vi "loadMSTReleaseFormNew.vi"() -> ()   [LabVIEW 2012]
uses:
  <vilib>/Utility/NIReport.llb/NI_report.lvclass
  <vilib>/addons/database/Connection.llb/DB Tools Open Connec (Path).vi
  <vilib>/addons/_office/excel.llb/Excel Get Data (str).vi
  <vilib>/addons/database/Connection.llb/Conn Execute.vi
  <vilib>/addons/database/Recordset.llb/Rec Fetch Integer Data (R).vi
  <vilib>/addons/database/Recordset.llb/Rec Destroy - Connection.vi
  <vilib>/Utility/NIReport.llb/Excel/NI_Excel.lvclass
  <vilib>/addons/_office/NI_ReportGenerationToolkit.lvlib
  <vilib>/addons/database/NI_Database_API.lvlib
panel:
  out "data 2":i32
  out "appended path 4":path
  out "appended path 3":path
  out "concatenated string 3":string
  out "error out 3":errorcluster
  out "row":i32
  out "concatenated string 2":string
  out "appended path 2":path
  out "data":string
  in  "start (0, 0)":cluster{"start row":i32, "start column":i32}
  out "PCB":string
  out "TestProgram":string
  out "Temp":string
  out "Product":string
  out "x+y":dbl
  out "String":string
  out "error out":errorcluster
  out "concatenated string":string
  out "error out 4":errorcluster
  out "appended path":path
  out "error out 2":errorcluster
  in  "path":path=path "O:/Monitor/Recipe/MST"
  out "filenames":string[](array[string])
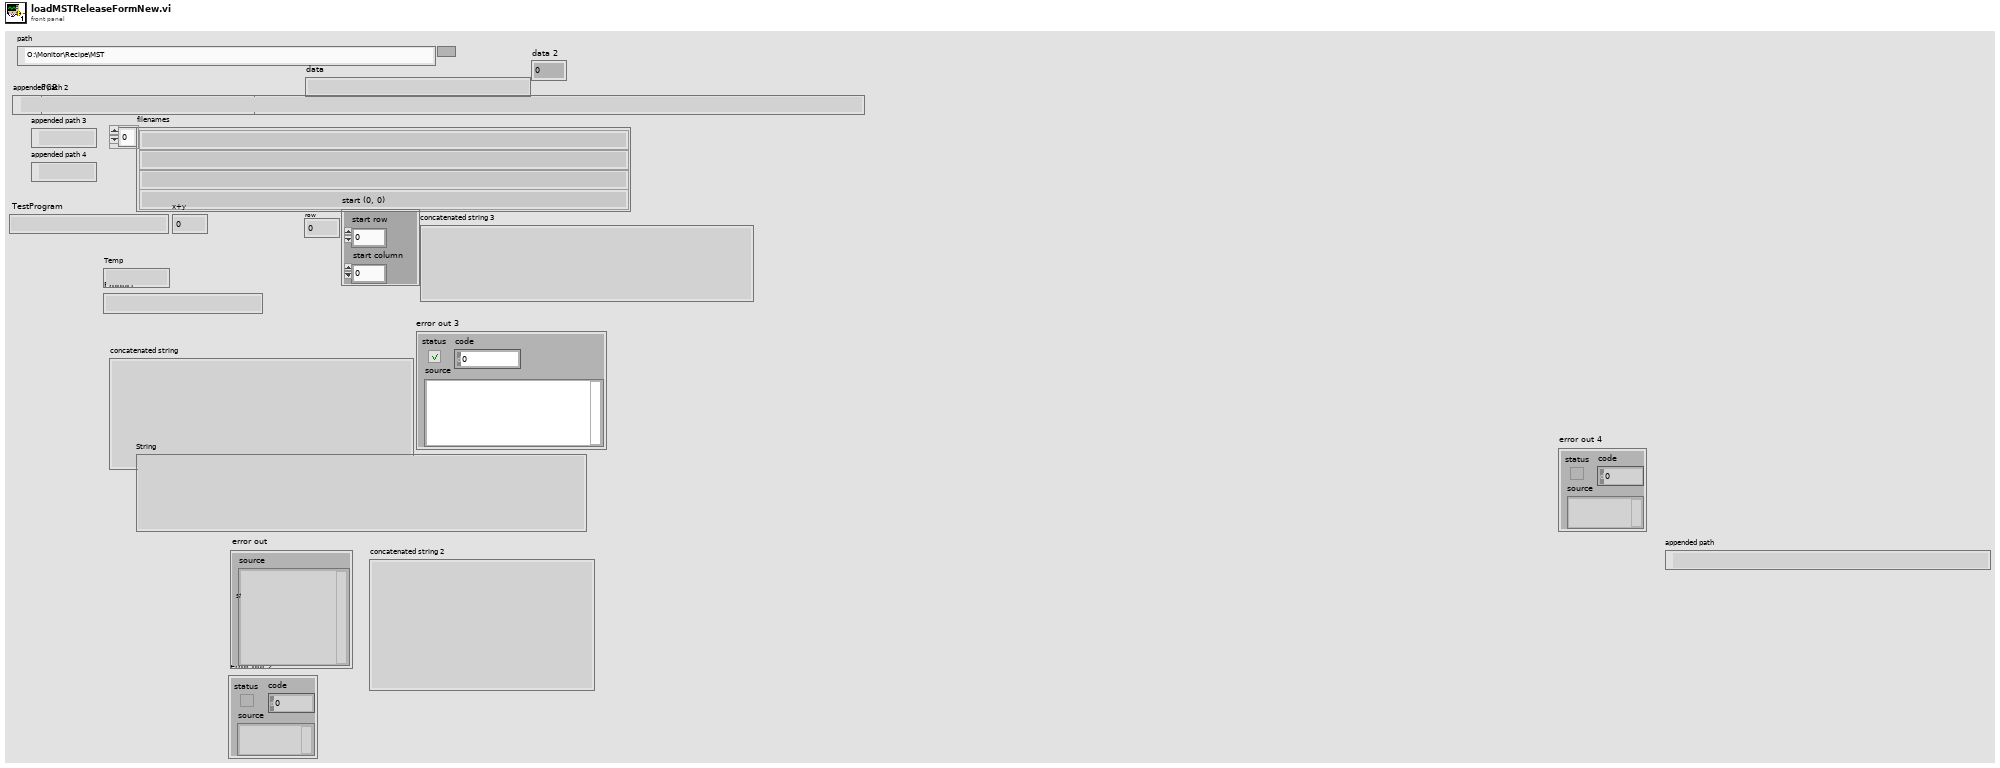
[diagram p1: front panel]
types:
  T1 = enum16{"Standard Report", "HTML", "Word", "Excel"}
  T2 = typedef "NI_Database_API.lvlib/Conn ObjectReference.ctl" = refnum<k1>
  T3 = typedef "NI_Database_API.lvlib/Rec ObjectReference.ctl" = refnum<k1>
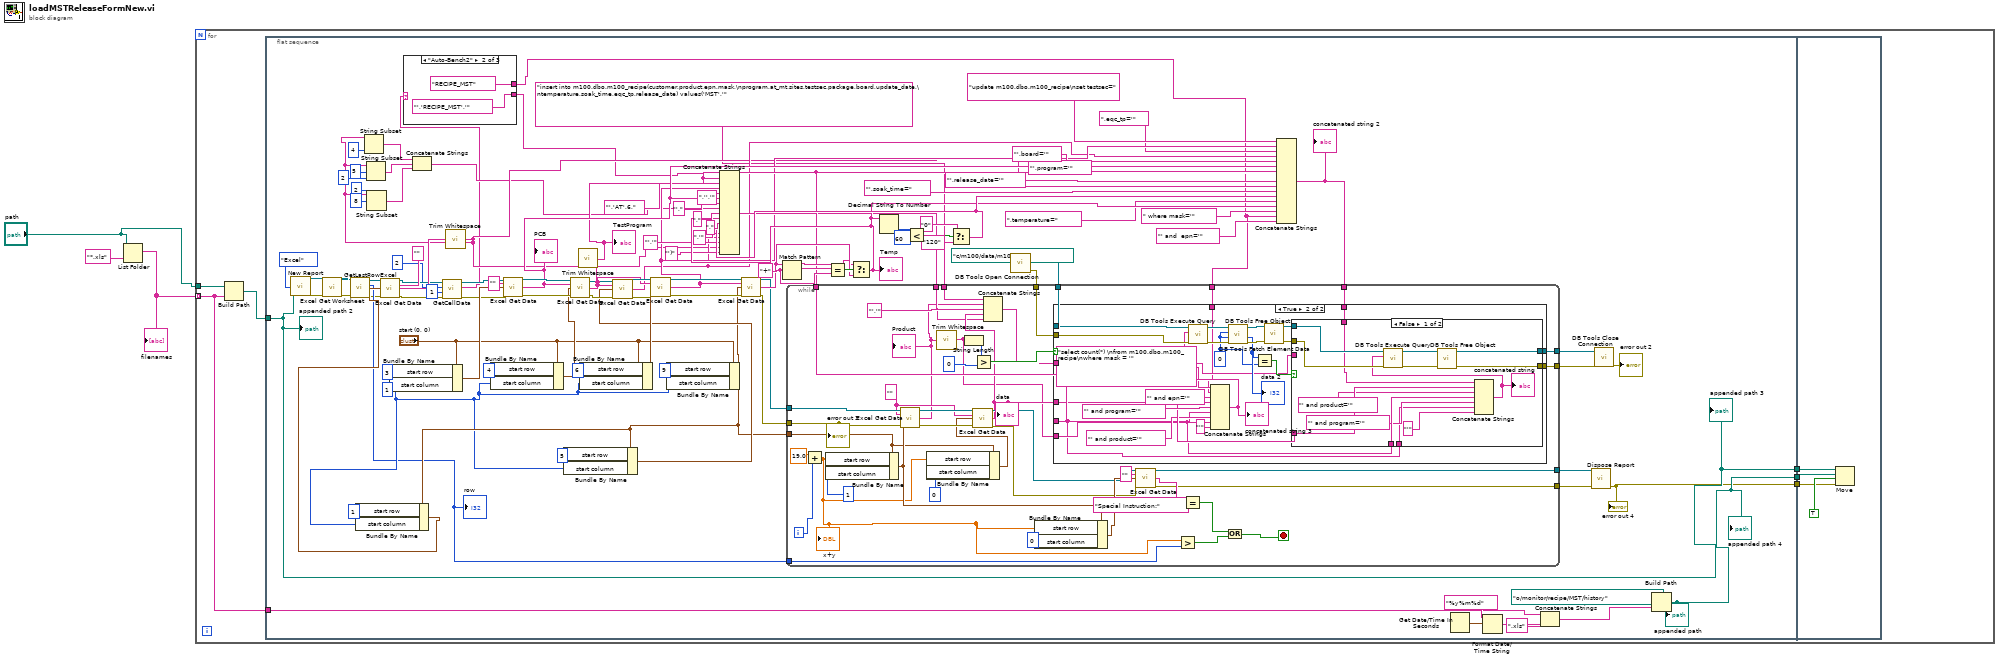
[diagram p0: block diagram]
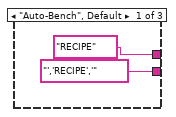
[diagram p2: hidden frame]
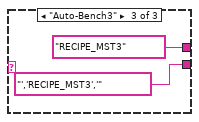
[diagram p3: hidden frame]
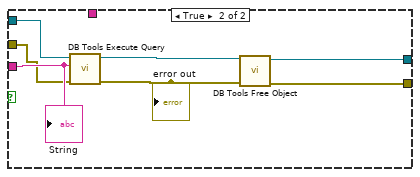
[diagram p5: hidden frame]
diagram:
  n1 = List Folder(path="path", pattern="*.xls") -> (filenames=w1:string[])  [unwired: 2 in, 3 out]
  "filenames" <- w1
  n2 = for {
    tunnel: "path" -> [w9]
    tunnel: w1 -> [w8] mode=indexing
    n3 = Build Path(base path=w9, name or relative path=w8) -> (appended path=w5:path)
    n4 = flat-sequence {
      tunnel: w8 -> [w74]
      tunnel: [w35] -> w7
      tunnel: [w34] -> w6
      tunnel: w5 -> [w34]
      tunnel: [w23] -> w4
      tunnel: w7 -> [w218]
      tunnel: w6 -> [w219]
      tunnel: w4 -> [w216]
      frame #0 {
        w101 = "+" ("regular expression")
        w48 = 1 ("start column")
        n5 = call <vilib>:"New Report.vi"("report type"=T1."Excel" ("Report Type"), "template (empty)"=w34) -> ("report out"=w117:refnum<class "NI_report.lvclass">, "error out"=w116:errorcluster)  [unwired: 12 in]
        n6 = call <vilib>:"Excel Get Worksheet.vi"("report in"=w117, "error in (no error)"=w116) -> ("report out"=w42:refnum<class "NI_report.lvclass">, "error out"=w43:errorcluster)  [unwired: 12 in]
        n7 = call "GetLastRowExcel.vi"("error in (no error)"=w43, "report in"=w42) -> ("error out"=w21:errorcluster, "row"=w40:i32, "report out"=w41:refnum<class "NI_report.lvclass">)  [unwired: 7 in]
        "row" <- w40
        n8 = Bundle By Name(cluster="start (0, 0)", "start row"=3, "start column"=w48) -> (w115:cluster{"start row":i32, "start column":i32})
        n9 = Bundle By Name(cluster="start (0, 0)", "start row"=4, "start column"=w48) -> (w109:cluster{"start row":i32, "start column":i32})
        n10 = Bundle By Name(cluster="start (0, 0)", "start row"=6, "start column"=w48) -> (w107:cluster{"start row":i32, "start column":i32})
        n11 = Bundle By Name(cluster="start (0, 0)", "start row"=9, "start column"=w48) -> (w49:cluster{"start row":i32, "start column":i32})
        n12 = Bundle By Name(cluster=w49, "start row"=1, "start column"=w48) -> (w47:cluster{"start row":i32, "start column":i32})
        n13 = call-poly <vilib>:"Excel Get Data.vi"("report in"=w41, "data type"="", "start (0, 0)"=w47, "error in (no error)"=w21) -> ("report out"=w22:refnum<class "NI_report.lvclass">, "data"=w44:string, "error out"=w20:errorcluster)  [unwired: 9 in]
        n14 = call "GetCellData.vi"("error in (no error)"=w20, "start column"=1, "start row"=2, "report in"=w22) -> ("error out"=w17:errorcluster, "data"=w15:string, "report out"=w16:refnum<class "NI_report.lvclass">)  [unwired: 5 in]
        n15 = case shown="\"Auto-Bench2\"" w15 {
          tunnel: ["','RECIPE','" ("string") "','RECIPE_MST','" ("string") "','RECIPE_MST3','" ("string")] -> w11
          tunnel: ["RECIPE" "RECIPE_MST" "RECIPE_MST3"] -> w10
          frame "Auto-Bench", Default {
          }
          frame "Auto-Bench2" {
          }
          frame "Auto-Bench3" {
          }
        }
        n16 = call <vilib>:"Trim Whitespace.vi"("string"=w44) -> ("trimmed string"=w30:string)  [unwired: 1 in]
        n17 = String Subset(string=w30, length (rest)=4 ("length (rest)")) -> (substring=w27:string)  [unwired: 1 in]
        n18 = String Subset(string=w30, offset (0)=5, length (rest)=2 ("length (rest)")) -> (substring=w26:string)
        n19 = String Subset(string=w30, offset (0)=8, length (rest)=2 ("length (rest)")) -> (substring=w25:string)
        n20 = Concatenate Strings(w27, w26, w25) -> (w24:string)
        n21 = call-poly <vilib>:"Excel Get Data.vi"("report in"=w16, "data type"="", "start (0, 0)"=w115, "error in (no error)"=w17) -> ("report out"=w111:refnum<class "NI_report.lvclass">, "data"=w84:string, "error out"=w112:errorcluster)  [unwired: 9 in]
        "PCB" <- w84
        n22 = Bundle By Name(cluster=w49, "start row"=5, "start column"=w48) -> (w53:cluster{"start row":i32, "start column":i32})
        n23 = call-poly <vilib>:"Excel Get Data.vi"("report in"=w111, "data type"=w84, "start (0, 0)"=w109, "error in (no error)"=w112) -> ("report out"=w59:refnum<class "NI_report.lvclass">, "data"=w55:string, "error out"=w57:errorcluster)  [unwired: 9 in]
        n24 = call <vilib>:"Trim Whitespace.vi"("string"=w55) -> ("trimmed string"=w61:string)  [unwired: 1 in]
        "TestProgram" <- w61
        n25 = call-poly <vilib>:"Excel Get Data.vi"("report in"=w59, "data type"=w55, "start (0, 0)"=w53, "error in (no error)"=w57) -> ("report out"=w58:refnum<class "NI_report.lvclass">, "data"=w36:string, "error out"=w56:errorcluster)  [unwired: 9 in]
        n26 = call-poly <vilib>:"Excel Get Data.vi"("report in"=w58, "data type"=w55, "start (0, 0)"=w107, "error in (no error)"=w56) -> ("report out"=w104:refnum<class "NI_report.lvclass">, "data"=w38:string, "error out"=w105:errorcluster)  [unwired: 9 in]
        n27 = call-poly <vilib>:"Excel Get Data.vi"("report in"=w104, "data type"=w38, "start (0, 0)"=w49, "error in (no error)"=w105) -> ("report out"=w97:refnum<class "NI_report.lvclass">, "data"=w99:string, "error out"=w96:errorcluster)  [unwired: 9 in]
        n28 = Match Pattern(string=w99, regular expression=w101) -> (before substring=w98:string, match substring=w102:string)  [unwired: 1 in, 2 out]
        n29 = Equal?(x=w102, y=w101) -> (x = y?=w100:bool)
        n30 = Select(t=w98, s=w100, f=w99) -> (s? t:f=w63:string)
        "Temp" <- w63
        n31 = Decimal String To Number(string=w63) -> (number=w70:i32)  [unwired: 2 in, 1 out]
        n32 = Less?(x=w70, y=60) -> (x < y?=w68:bool)
        n33 = Select(t="0", s=w68, f="120") -> (s? t:f=w64:string)
        n34 = Concatenate Strings(w11, w61, "','AT',6," ("string"), w38, ",'','" ("string"), w84, "'," ("string"), w24, "," ("string"), w63, "," ("string"), w64, ",'" ("string"), w36, "','" ("string"), w30, "')" ("string")) -> (w60:string)
        n35 = call-poly <vilib>:"DB Tools Open Connection.vi"("connection information"=path "c:/m100/data/m100.dsn") -> ("error out"=w94:errorcluster, "connection reference"=w95:T2)  [unwired: 7 in]
        n36 = Concatenate Strings("update m100.dbo.m100_recipe\nset testsec=", w38, ",eqc_tp='" ("string"), w36, "',board='" ("string"), w84, "',program='" ("string"), w61, "',release_date='" ("string"), w30, "',soak_time=" ("string"), w64, ",temperature=" ("string"), w63, " where mask='" ("string"), w10, "' and  epn='" ("string")) -> (w81:string)
        "concatenated string 2" <- w81
        n37 = while {
          tunnel: w97 -> [w167]
          tunnel: w96 -> [w166]
          tunnel: w49 -> [w139]
          tunnel: w95 -> [w153]
          tunnel: w94 -> [w152]
          tunnel: "insert into m100.dbo.m100_recipe(customer,product,epn,mask,\nprogram,at_mt,sites,testsec,package,board,update_date,\ntemperature,soak_time,eqc_tp,release_date) values('MST','" ("string") -> [w136]
          tunnel: w60 -> [w133]
          tunnel: [w150] -> w89
          tunnel: [w149] -> w88
          tunnel: [w148] -> w87
          tunnel: [w147] -> w86
          tunnel: w81 -> [w146]
          tunnel: w61 -> [w137]
          tunnel: w40 -> [w128]
          tunnel: w10 -> [w125]
          i -> [w161]
          stop <- w130 stop-if-true
          w141 = "" ("data type")
          n38 = Add(x=19.0, y=w161) -> (x+y=w132:dbl)
          "x+y" <- w132
          n39 = Bundle By Name(cluster=w139, "start row"=w132, "start column"=1) -> (w158:cluster{"start row":i32, "start column":i32})
          n40 = call-poly <vilib>:"Excel Get Data.vi"("report in"=w167, "data type"=w141, "start (0, 0)"=w158, "error in (no error)"=w166) -> ("report out"=w143:refnum<class "NI_report.lvclass">, "data"=w127:string, "error out"=w142:errorcluster)  [unwired: 9 in]
          "Product" <- w127
          n41 = Bundle By Name(cluster=w139, "start row"=w132, "start column"=0) -> (w138:cluster{"start row":i32, "start column":i32})
          n42 = call <vilib>:"Trim Whitespace.vi"("string"=w127) -> ("trimmed string"=w126:string)  [unwired: 1 in]
          n43 = String Length(string=w126) -> (length=w164:i32)
          n44 = call-poly <vilib>:"Excel Get Data.vi"("report in"=w143, "data type"=w141, "start (0, 0)"=w138, "error in (no error)"=w142) -> ("report out"=w145:refnum<class "NI_report.lvclass">, "data"=w134:string, "error out"=w144:errorcluster)  [unwired: 9 in]
          "data" <- w134
          n45 = Greater?(x=w164, y=0) -> (0:w154:bool)
          n46 = Concatenate Strings(w136, w127, "','" ("string"), w134, w133) -> (w151:string)
          n47 = Bundle By Name(cluster=w158, "start row"=w132, "start column"=0) -> (w159:cluster{"start row":i32, "start column":i32})
          n48 = case shown="True" w154 {
            tunnel: w153 -> [w169 w194]
            tunnel: w152 -> [w168 w193]
            tunnel: w134 -> [_ w177]
            tunnel: w151 -> [_ w179]
            tunnel: [w169 w181] -> w150
            tunnel: [w168 w180] -> w149
            tunnel: w146 -> [_ w178]
            tunnel: w137 -> [_ w173]
            tunnel: w126 -> [_ w174]
            tunnel: w125 -> [_ w171]
            frame False {
            }
            frame True {
              w185 = 0
              n49 = Concatenate Strings("select count(*) \nfrom m100.dbo.m100_recipe\nwhere mask = '" ("string"), w171, "' and epn='" ("string"), w177, "' and program='" ("string"), w173, "' and product='" ("string"), w174, "'" ("string")) -> (w191:string)
              "concatenated string 3" <- w191
              n50 = call-poly <vilib>:"DB Tools Execute Query.vi"("error in (no error)"=w193, "SQL query"=w191, "connection reference"=w194) -> ("error out"=w189:errorcluster, "recordset reference"=w190:T3)  [unwired: 5 in]
              n51 = call-poly <vilib>:"DB Tools Fetch Element Data.vi"("error in (no error)"=w189, "type"=w185, "column index"=w185, "recordset reference"=w190) -> ("error out"=w187:errorcluster, "data"=w186:i32, "recordset reference out"=w188:T3)  [unwired: 3 in]
              "data 2" <- w186
              n52 = Equal?(x=w186, y=w185) -> (x = y?=w184:bool)
              n53 = call-poly <vilib>:"DB Tools Free Object.vi"("error in (no error)"=w187, "recordset reference"=w188) -> ("error out"=w182:errorcluster, "connection reference"=w183:T2)  [unwired: 8 in]
              n54 = case shown="False" w184 {
                tunnel: w179 -> [_ w215]
                tunnel: w183 -> [w208 w214]
                tunnel: w182 -> [w207 w213]
                tunnel: [w204 w210] -> w181
                tunnel: [w203 w209] -> w180
                tunnel: w178 -> [w202 _]
                tunnel: w177 -> [w201 _]
                tunnel: w174 -> [w198 _]
                tunnel: w173 -> [w196 _]
                frame False {
                  n55 = Concatenate Strings(w202, w201, "' and product='" ("string"), w198, "' and program='" ("string"), w196, "'" ("string")) -> (w199:string)
                  "concatenated string" <- w199
                  n56 = call-poly <vilib>:"DB Tools Execute Query.vi"("error in (no error)"=w207, "SQL query"=w199, "connection reference"=w208) -> ("error out"=w205:errorcluster, "recordset reference"=w206:T3)  [unwired: 5 in]
                  n57 = call-poly <vilib>:"DB Tools Free Object.vi"("error in (no error)"=w205, "recordset reference"=w206) -> ("error out"=w203:errorcluster, "connection reference"=w204:T2)  [unwired: 8 in]
                }
                frame True {
                  n58 = call-poly <vilib>:"DB Tools Execute Query.vi"("error in (no error)"=w213, "SQL query"=w215, "connection reference"=w214) -> ("error out"=w212:errorcluster, "recordset reference"=w211:T3)  [unwired: 5 in]
                  "error out" <- w212
                  n59 = call-poly <vilib>:"DB Tools Free Object.vi"("error in (no error)"=w212, "recordset reference"=w211) -> ("error out"=w209:errorcluster, "connection reference"=w210:T2)  [unwired: 8 in]
                  "String" <- w215
                }
              }
            }
          }
          n60 = call-poly <vilib>:"Excel Get Data.vi"("report in"=w145, "data type"="", "start (0, 0)"=w159, "error in (no error)"=w144) -> ("report out"=w148:refnum<class "NI_report.lvclass">, "data"=w156:string, "error out"=w147:errorcluster)  [unwired: 9 in]
          n61 = Greater?(x=w132, y=w128) -> (0:w129:bool)
          n62 = Equal?(x=w156, y="Special Instruction:") -> (x = y?=w131:bool)
          n63 = Or(x=w131, y=w129) -> (x .or. y?=w130:bool)
          "error out 3" <- w166
        }
        n64 = Get Date/Time In Seconds() -> (seconds since 1Jan1904=w78:timestamp)
        n65 = Format Date/Time String(time format string (%c)="%y%m%d", seconds (now)=w78) -> (date/time string=w76:string)  [unwired: 1 in]
        n66 = Concatenate Strings(w74, w76, ".xls" ("string")) -> (w79:string)
        n67 = call-dynamic "Dispose Report.vi"("report in"=w87, "error in (no error)"=w86) -> ("error out"=w23:errorcluster)  [unwired: 13 in]
        "error out 4" <- w23
        n68 = call <vilib>:"DB Tools Close Connection.vi"("error in (no error)"=w88, "connection reference"=w89) -> ("error out"=→"error out 2":errorcluster)  [unwired: 5 in]
        n69 = Build Path(base path=path "o:/monitor/recipe/MST/history", name or relative path=w79) -> (appended path=w35:path)
        "appended path" <- w35
        "appended path 4" <- w35
        "appended path 2" <- w34
        "appended path 3" <- w34
      }
      frame #1 {
        n70 = Move(source path=w219, error in=w216, 9:TRUE ("overwrite (F)"), 10:w218) -> ()  [unwired: 1 in, 3 out]
      }
    }
  }
